vi "dlgSelectVisApps.vi"(8 "Error In":errorcluster[](array[cluster])) -> (0 "Error Out":errorcluster[](array[cluster]))   [LabVIEW 2017, in "Framework.lvlib"]
uses:
  Framework.lvlib
  <userlib>/NIST/NISTErrorLib/NISTErrorLib.lvlib
panel:
  in  "btnRun":bool
  in  "btnCancel":bool
  in  "selArray":cluster{"chkSelect":bool, "strVis":string}[](array[cluster]) caption="Select Visualization Apps"
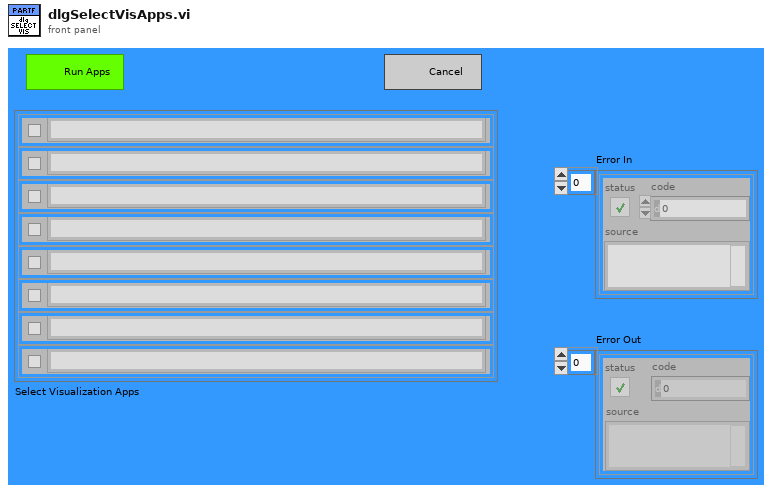
[diagram p1: front panel]
types:
  T1 = typedef "Framework.lvlib/clFrontPanelControlRefs.ctl" = cluster{"TestFilePathRef":refnum<vi>, "BusNumberRef":refnum<vi>, "NumberOfBusesRef":refnum<vi>, "EvtTypeRef":refnum<vi>, "EvtParamsRef":refnum<vi>, "EvtConfigRef":refnum<vi>, "StartTimeRef":refnum<vi>, "EndTimeRef":refnum<vi>, "PmuImpairTypeRef":refnum<vi>, "PmuImpairParamsRef":refnum<vi>, "NetImpairParamsRef":refnum<vi>, "FlagImpairTypeRef":refnum<vi>, "FlagImpairParamsRef":refnum<vi>, "NetImpairTypeRef":refnum<vi>, "OutputFileType":refnum<vi>, "PmuImpairConfigRef":refnum<vi>, "AppTypeRef":refnum<vi>, "ScriptPathRef":refnum<vi>, "ShowPanels?":refnum<vi>}
  T2 = typedef "LVRectTypeDef.ctl" = cluster{"Left":i16, "Top":i16, "Right":i16, "Bottom":i16}
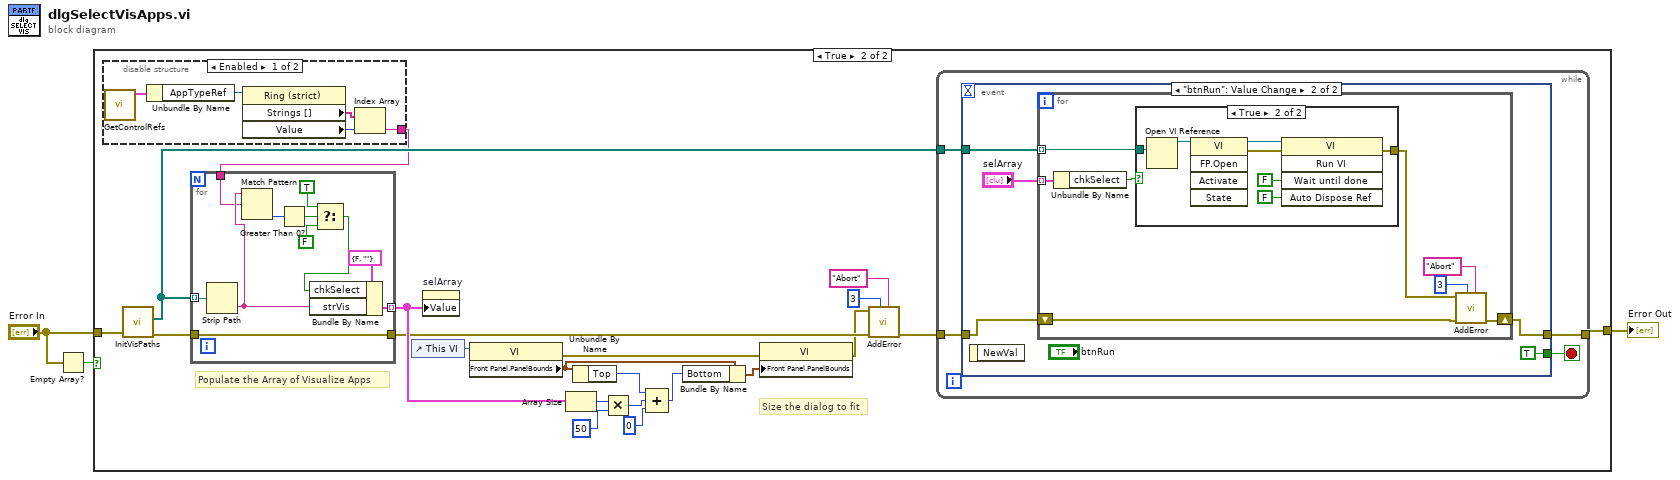
[diagram p0: block diagram]
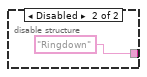
[diagram p3: hidden frame]
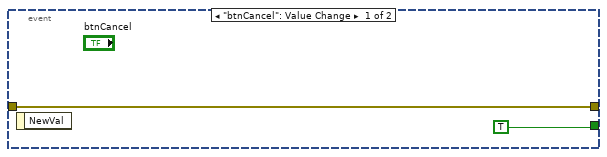
[diagram p4: hidden frame]
diagram:
  n1 = Empty Array?(array="Error In") -> (empty?=w3:bool)
  n2 = case shown="True" w3 {
    tunnel: "Error In" -> [w4 w25]
    tunnel: [w4 w23] -> w1
    frame False {
    }
    frame True {
      # "Size the dialog to fit"
      # "Populate the Array of Visualize Apps"
      n3 = disable-structure shown="Enabled" {
        disable-tunnel: [w30 "Ringdown"] -> w20
        frame Enabled {
          n4 = call "GetControlRefs.vi"() -> ("clControlRefs Out"=w29:T1)  [unwired: 11 in]
          n5 = Unbundle By Name(w29) -> ("AppTypeRef"=w28:refnum<vi>)
          n6 = property class="Ring (strict)"(reference=w28) -> ("Strings []"=w26:string[], "Value"=w27:u16)  [unwired: 1 in, 2 out]
          n7 = Index Array(array=w26, index=w27) -> (element=w30:string)
        }
        frame Disabled {
        }
      }
      n8 = call "InitVisPaths.vi"("ErrorArray In"=w25) -> ("ErrorArray Out"=w24:errorcluster[], "VisualizeFilePaths"=w21:path[])  [unwired: 9 in]
      n9 = for {
        tunnel: w21 -> [w39] mode=indexing
        tunnel: [w41] -> w22 mode=indexing
        tunnel: w24 -> [w40]
        tunnel: [w40] -> w11
        tunnel: w20 -> [w37]
        n10 = Strip Path(path=w39) -> (name=w38:string)  [unwired: 1 out]
        n11 = Match Pattern(string=w38, regular expression=w37) -> (offset past match=w36:i32)  [unwired: 1 in, 3 out]
        n12 = Greater Than 0?(x=w36) -> (x > 0?=w35:bool)
        n13 = Select(t=TRUE, s=w35, f=FALSE) -> (s? t:f=w34:bool)
        n14 = Bundle By Name(cluster=cluster{"chkSelect":bool, "strVis":string} {"chkSelect"=FALSE, "strVis"=""} ("elementSelArray"), "chkSelect"=w34, "strVis"=w38) -> (w41:cluster{"chkSelect":bool, "strVis":string})
      }
      n15 = control-ref of="This VI"() -> (w12:refnum<vi>)
      n16 = property on="selArray" class="Arr (strict)"("Value"=w22) -> ()  [unwired: 2 in, 2 out]
      n17 = property class="VI"(reference=w12) -> (error out=w13:errorcluster, "Front Panel.PanelBounds"=w6:T2)  [unwired: 1 in, 1 out]
      n18 = Array Size(array=w22) -> (size(s)=w14:i32)
      n19 = Unbundle By Name(w6) -> ("Top"=w5:i16)
      n20 = Multiply(x=w14, y=50 ("x")) -> (x*y=w16:i32)
      n21 = Compound Arithmetic op=ADD(w5, w16, 0 ("x")) -> (w19:i32)
      n22 = Bundle By Name(cluster=w6, "Bottom"=w19) -> (w18:T2)
      n23 = property class="VI"(error in=w13, "Front Panel.PanelBounds"=w18) -> (error out=w9:errorcluster)  [unwired: 1 in, 1 out]
      n24 = call <userlib>:"AddError.vi"("Severity"="Abort", "Priority"=u8 3, "ErrorArray"=w11, "error in (no error)"=w9) -> ("ErrorArray"=w10:errorcluster[])  [unwired: 6 in, 1 out]
      n25 = while {
        tunnel: w10 -> [w45]
        tunnel: [w44] -> w23
        tunnel: w21 -> [w43]
        stop <- w46 stop-if-true
        n26 = event shown="[1] \"btnRun\": Value Change" {
          selector: _ -> [_ _]
          dyn-events: _ -> [_ _]
          timeout: _ -> [_ _]
          tunnel: [TRUE TRUE] -> w46
          tunnel: [w47 w49] -> w44
          tunnel: w45 -> [w47 w50]
          tunnel: w43 -> [_ w52]
          event "btnCancel": Value Change {
            n27 = event-data() -> ()  [unwired: 1 in, 1 out]
          }
          event "btnRun": Value Change {
            n28 = event-data() -> ()  [unwired: 1 in, 1 out]
            n29 = for {
              tunnel: "selArray" -> [w61] mode=indexing
              tunnel: w52 -> [w59] mode=indexing
              shift-right: [w58] -> w49
              shift-left: w50 -> [w54]
              n30 = Unbundle By Name(w61) -> ("chkSelect"=w60:bool)
              n31 = case shown="True" w60 {
                tunnel: w59 -> [_ w63]
                tunnel: [_ w62] -> w57
                frame False {
                }
                frame True {
                  n32 = Open VI Reference(vi path=w63) -> (vi reference=w68:refnum<vi>)  [unwired: 5 in, 1 out]
                  n33 = invoke class="VI" method="FP.Open"(reference=w68) -> (reference out=w65:refnum<vi>, error out=w64:errorcluster)  [unwired: 4 in, 3 out]
                  n34 = invoke class="VI" method="Run VI"(reference=w65, error in=w64, "Wait until done"=FALSE ("Wait Until Done"), "Auto Dispose Ref"=FALSE ("Auto Dispose Reference")) -> (error out=w62:errorcluster)  [unwired: 1 in, 4 out]
                }
              }
              n35 = call <userlib>:"AddError.vi"("Severity"="Abort", "Priority"=u8 3, "ErrorArray"=w54, "error in (no error)"=w57) -> ("ErrorArray"=w58:errorcluster[])  [unwired: 6 in, 1 out]
            }
          }
        }
      }
    }
  }
  "Error Out" <- w1
